vi "Open.vi"   [LabVIEW 2014, in "MBUG-2820.lvlib"]
doc: "Open a device by its id string (MBUG-2820-XXXXXX) or its serial number (last 6 digits of the id string).\nReturns a device handle, that must be passed to the functions accessing the deivce."
uses:
  <instrlib>/MBUG-2820/MBUG-2820.lvlib
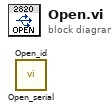
[diagram p0: block diagram]
diagram:
  n1 = call <instrlib>:"Open_serial.vi"() -> ()  [unwired: 6 in, 2 out]
  n2 = call <instrlib>:"Open_id.vi"() -> ()  [unwired: 6 in, 2 out]
